vi "SaveFile.vi"(8 "error in (no error)":errorcluster, 9 "Sound Format":T1={"sample rate (S/s)"=22050.0, "number of channels"=2, "bits per sample"=16}, 10 "Waveform(s) in":waveform(dbl)[](array[waveform])) -> (0 "error out":errorcluster)   [LabVIEW 2019]
uses:
  <vilib>/sound2/lvsound2.llb/Sound File Write Open.vi
  <vilib>/sound2/lvsound2.llb/Sound File Write (DBL).vi
  <vilib>/sound2/lvsound2.llb/Sound Data Format.ctl
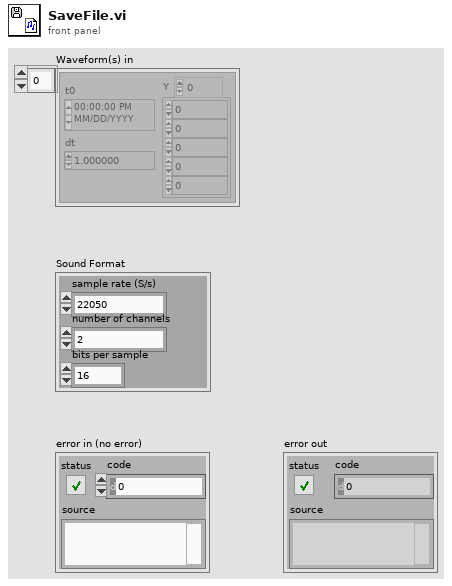
[diagram p1: front panel]
types:
  T1 = typedef "Sound Data Format.ctl" = cluster{"sample rate (S/s)":dbl, "number of channels":i32, "bits per sample":i32}
  T2 = typedef "Sound File Refnum.ctl" = refnum<file>
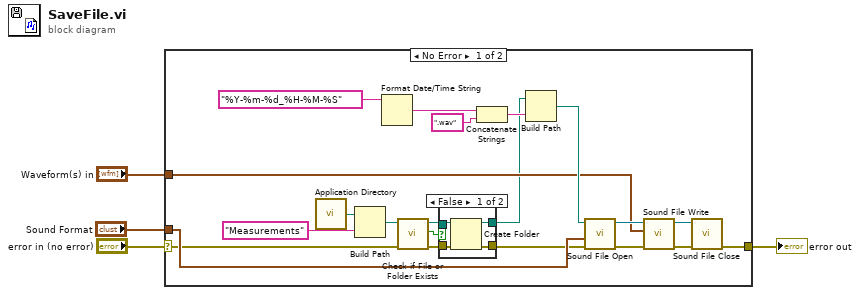
[diagram p0: block diagram]
diagram:
  n1 = case shown="No Error" "error in (no error)" {
    selector: "error in (no error)" -> [w11 w32]
    tunnel: [w17 w32] -> w4
    tunnel: "Waveform(s) in" -> [w13 _]
    tunnel: "Sound Format" -> [w12 _]
    frame No Error {
      n2 = call <vilib>:"Application Directory.vi"() -> ("Application Directory"=w14:path)
      n3 = Build Path(base path=w14, name or relative path="Measurements") -> (appended path=w7:path)
      n4 = Format Date/Time String(time format string (%c)="%Y-%m-%d_%H-%M-%S") -> (date/time string=w22:string)  [unwired: 2 in]
      n5 = call <vilib>:"Check if File or Folder Exists.vi"("error in (no error)"=w11, "path"=w7) -> ("error out"=w10:errorcluster, "file or folder exists?"=w6:bool, "dup path"=w8:path)  [unwired: 7 in]
      n6 = case shown="False" w6 {
        tunnel: w10 -> [w29 w30]
        tunnel: [w28 w30] -> w9
        tunnel: w8 -> [w27 w31]
        tunnel: [w26 w31] -> w5
        frame False {
          n7 = Create Folder(path (use dialog)=w27, error in=w29) -> (created path=w26:path, error out=w28:errorcluster)  [unwired: 1 in, 1 out]
        }
        frame True {
        }
      }
      n8 = Concatenate Strings(w22, ".wav" ("string")) -> (w24:string)
      n9 = Build Path(base path=w5, name or relative path=w24) -> (appended path=w16:path)
      n10 = call-poly <vilib>:"Sound File Open.vi"("error in (no error)"=w9, "sound format"=w12, "path"=w16) -> ("error out"=w20:errorcluster, "sound file refnum"=w21:T2)  [unwired: 7 in]
      n11 = call-poly <vilib>:"Sound File Write.vi"("error in (no error)"=w20, "data"=w13, "sound file refnum"=w21) -> ("error out"=w19:errorcluster, "sound file refnum out"=w18:T2)  [unwired: 7 in]
      n12 = call <vilib>:"Sound File Close.vi"("error in (no error)"=w19, "sound file refnum"=w18) -> ("error out"=w17:errorcluster)  [unwired: 9 in]
    }
    frame Error {
    }
  }
  "error out" <- w4
